vi "Client_Create.vi"(0 "reference in":refnum<class "Client.lvclass">, 2 "Rooms":T1, 5 "Error In":errorcluster) -> (14 "reference out":refnum<class "Client.lvclass">, 19 "Error Out":errorcluster)   [LabVIEW 2024, in "Client.lvclass"]
uses:
  Client.lvclass/Client.ctl
  Client.lvclass
  Systems/LightingSystem_class/LightingSystem.lvclass
  Systems/HeatingSystem_class/HeatingSystem.lvclass
  Facade_class/Facade.lvclass
  House/House_class/House.lvclass
  Systems/SecuritySystem_class/SecuritySystem.lvclass
  Systems/MusicSystem_class/MusicSystem.lvclass
  House/Room_class/Room.lvclass
  Systems/Type Defs/Rooms Cluster Array.ctl
panel:
  # "Connector Pane"
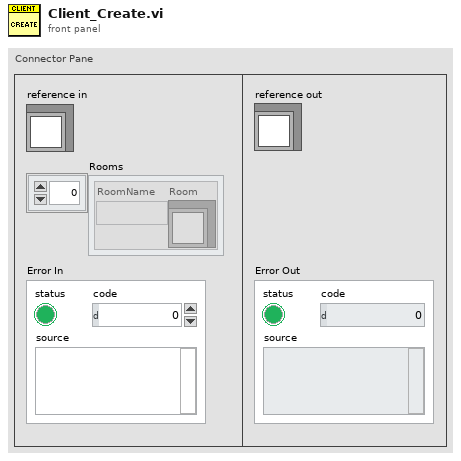
[diagram p1: front panel]
types:
  T1 = typedef "Rooms Cluster Array.ctl" = cluster{"RoomName":string, "Room":refnum<class "Room.lvclass">}[]
  T2 = typedef "Client.lvclass/ObjectAttributes.ctl" = cluster{"Facade":refnum<class "Facade.lvclass">}
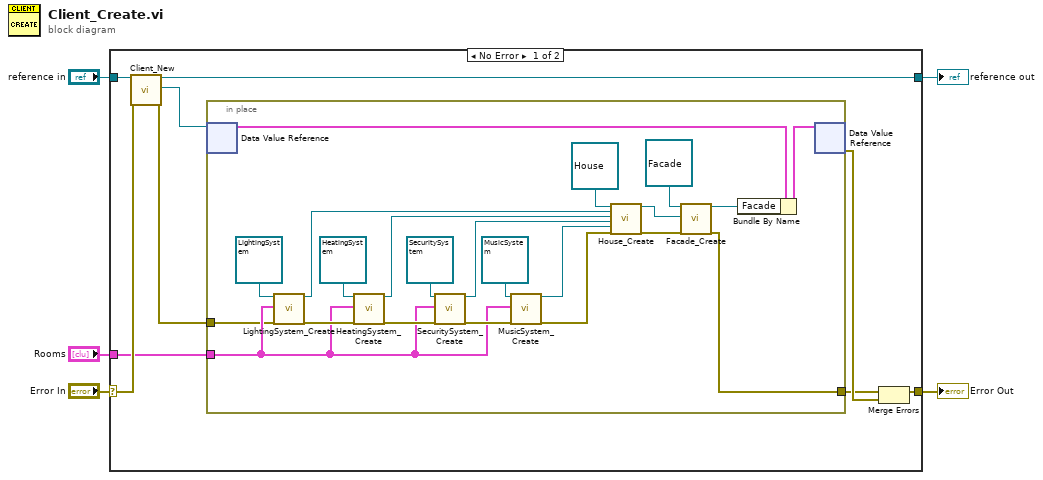
[diagram p0: block diagram]
diagram:
  n1 = case shown="No Error" "Error In" {
    selector: "Error In" -> [w13 w38]
    tunnel: [w10 w38] -> w4
    tunnel: "reference in" -> [w14 w37]
    tunnel: [w12 w37] -> w2
    tunnel: "Rooms" -> [w7 _]
    frame No Error {
      n2 = call "Client_New.vi"("reference in"=w14, "Error In"=w13) -> ("reference out"=w12:refnum<class "Client.lvclass">, "DVRRefOut"=w9:refnum<data-value>, "Error Out"=w6:errorcluster)  [unwired: 14 in, 1 out]
      n3 = in-place {
        in-place-border: [w15] -> w8
        in-place-border: w7 -> [w17]
        in-place-border: w6 -> [w16]
        n4 = in-place-dvr #1(w9) -> (w35:T2)  [unwired: 1 out]
        n5 = call "LightingSystem_Create.vi"("reference in"=refnum<class "LightingSystem.lvclass"> refnum ("LightingSystem"), "Rooms"=w17, "Error In"=w16) -> ("reference out"=w27:refnum<class "LightingSystem.lvclass">, "Error Out"=w34:errorcluster)  [unwired: 15 in]
        n6 = call "HeatingSystem_Create.vi"("reference in"=refnum<class "HeatingSystem.lvclass"> refnum ("HeatingSystem"), "Rooms"=w17, "Error In"=w34) -> ("reference out"=w26:refnum<class "HeatingSystem.lvclass">, "Error Out"=w25:errorcluster)  [unwired: 15 in]
        n7 = call "SecuritySystem_Create.vi"("reference in"=refnum<class "SecuritySystem.lvclass"> refnum ("SecuritySystem"), "Rooms"=w17, "Error In"=w25) -> ("reference out"=w24:refnum<class "SecuritySystem.lvclass">, "Error Out"=w28:errorcluster)  [unwired: 15 in]
        n8 = call "MusicSystem_Create.vi"("reference in"=refnum<class "MusicSystem.lvclass"> refnum ("MusicSystem"), "Rooms"=w17, "Error In"=w28) -> ("reference out"=w22:refnum<class "MusicSystem.lvclass">, "Error Out"=w23:errorcluster)  [unwired: 15 in]
        n9 = call "House_Create.vi"("reference in"=refnum<class "House.lvclass"> refnum ("House"), "Lighting System"=w27, "Heating System"=w26, "Security System"=w24, "Music System"=w22, "Error In"=w23) -> ("reference out"=w32:refnum<class "House.lvclass">, "Error Out"=w31:errorcluster)  [unwired: 12 in]
        n10 = call "Facade_Create.vi"("reference in"=refnum<class "Facade.lvclass"> refnum ("Facade"), "Home"=w32, "Error In"=w31) -> ("reference out"=w33:refnum<class "Facade.lvclass">, "Error Out"=w15:errorcluster)  [unwired: 15 in]
        n11 = Bundle By Name(cluster=w35, "Facade"=w33) -> (w36:T2)
        n12 = in-place-dvr #1(w36) -> (w11:errorcluster)  [unwired: 1 out]
      }
      n13 = Merge Errors(w8, w11) -> (w10:errorcluster)
    }
    frame Error {
      # "VI-TechBaseTemplate_Simple_6x8x6"
    }
  }
  "Error Out" <- w4
  "reference out" <- w2
